vi "PTv3.0.vi"(8 "error in":errorcluster) -> ()   [LabVIEW 2017]
doc: "This VI runs in parallel to other tasks. It can contain as many user-defined periodic loops as you need. These can carry out PID or other sorts of timed response."
uses:
  <vilib>/Analysis/baseanly.llb/Mean (DBL).vi
  <vilib>/Rock Robotics/WPI/Utilities/WPI_GetSetVariantRefNum.vi
  <vilib>/Rock Robotics/Network Tables/NT Read Boolean.vi
  Robot Global Data.vi
  <vilib>/Rock Robotics/Network Tables/NT Write Number.vi
  <vilib>/Rock Robotics/Network Tables/NT Write Numeric Array.vi
  <vilib>/Analysis/NI_AALBase.lvlib
panel:
  out "Arrayval":dbl
  out "Accelerations":T1
  out "Avg Y":dbl
  out "Current Joy Y Value":dbl
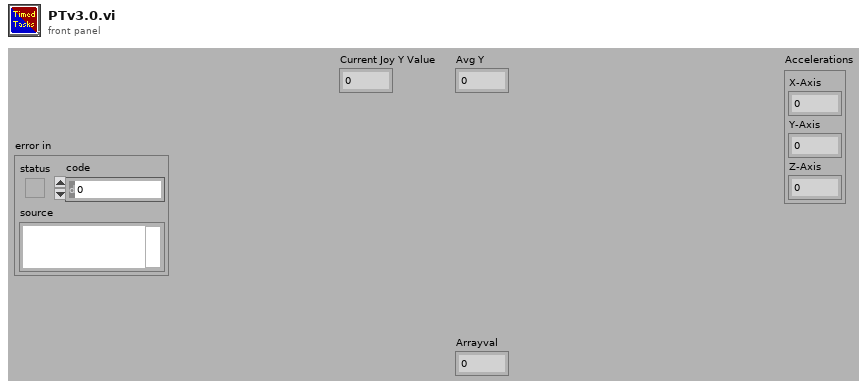
[diagram p1: front panel]
types:
  T1 = cluster{"X-Axis":dbl, "Y-Axis":dbl, "Z-Axis":dbl}
  T2 = typedef "WPI_JoystickDevRef.ctl" = cluster{"Device":T3}
  T3 = typedef "WPI_JoystickDeviceEnum.ctl" = enum16{"USB 0", "USB 1", "USB 2", "USB 3", "USB 4", "USB 5"}
  T4 = typedef "WPI_AccelerometerDevRef.ctl" = cluster{"DevStatus":errorcluster, "Scaling":T5, "Analog Channels":T6, "I2C Bus":T8, "SPI Bus":T9, "Accel Range":T10, "ADXL Axes":T11, "Handle":i32, "Device Address":u8, "Accel Type":enum16{"Analog", "ADXL345 I2C", "ADXL345 SPI", "Internal", "ADXL362 SPI"}}
  T5 = typedef "WPI_AccelerometerScaling.ctl" = cluster{"Gain (VoltsPerG)":dbl, "Center Voltage":dbl}
  T6 = typedef "WPI_AccelerometerAnalogChannels.ctl" = cluster{"X-Axis":T7, "Y-Axis":T7, "Z-Axis":T7}
  T7 = typedef "FPGA_AIChannel.ctl" = enum8{"AI 0", "AI 1", "AI 2", "AI 3", "AI MXP 0", "AI MXP 1", "AI MXP 2", "AI MXP 3", "Invalid"}
  T8 = typedef "i2c_bus.ctl" = enum16{"I2C On-Board", "I2C MXP", "Invalid"}
  T9 = typedef "spi_bus.ctl" = enum16{"SPI On-Board, CS0", "SPI On-Board, CS1", "SPI On-Board, CS2", "SPI On-Board, CS3", "SPI MXP", "Invalid"}
  T10 = typedef "ADXL345 Range.ctl" = u8
  T11 = typedef "WPI_AccelerometerADXL345 Axes.ctl" = cluster{"X-Axis":bool, "Y-Axis":bool, "Z-Axis":bool}
  T12 = typedef "WPI_GyroDevRef.ctl" = cluster{"DevStatus":errorcluster, "Analog Channel":T7, "Gain (VoltsPerDegree/Second)":dbl, "Gyro Type":enum16{"Analog", "XRS450"}, "Handle":i32, "SPI Bus":T9, "Device Found":bool, "Sample Rate":dbl, "Calibrate On Open":bool, "Offset":dbl}
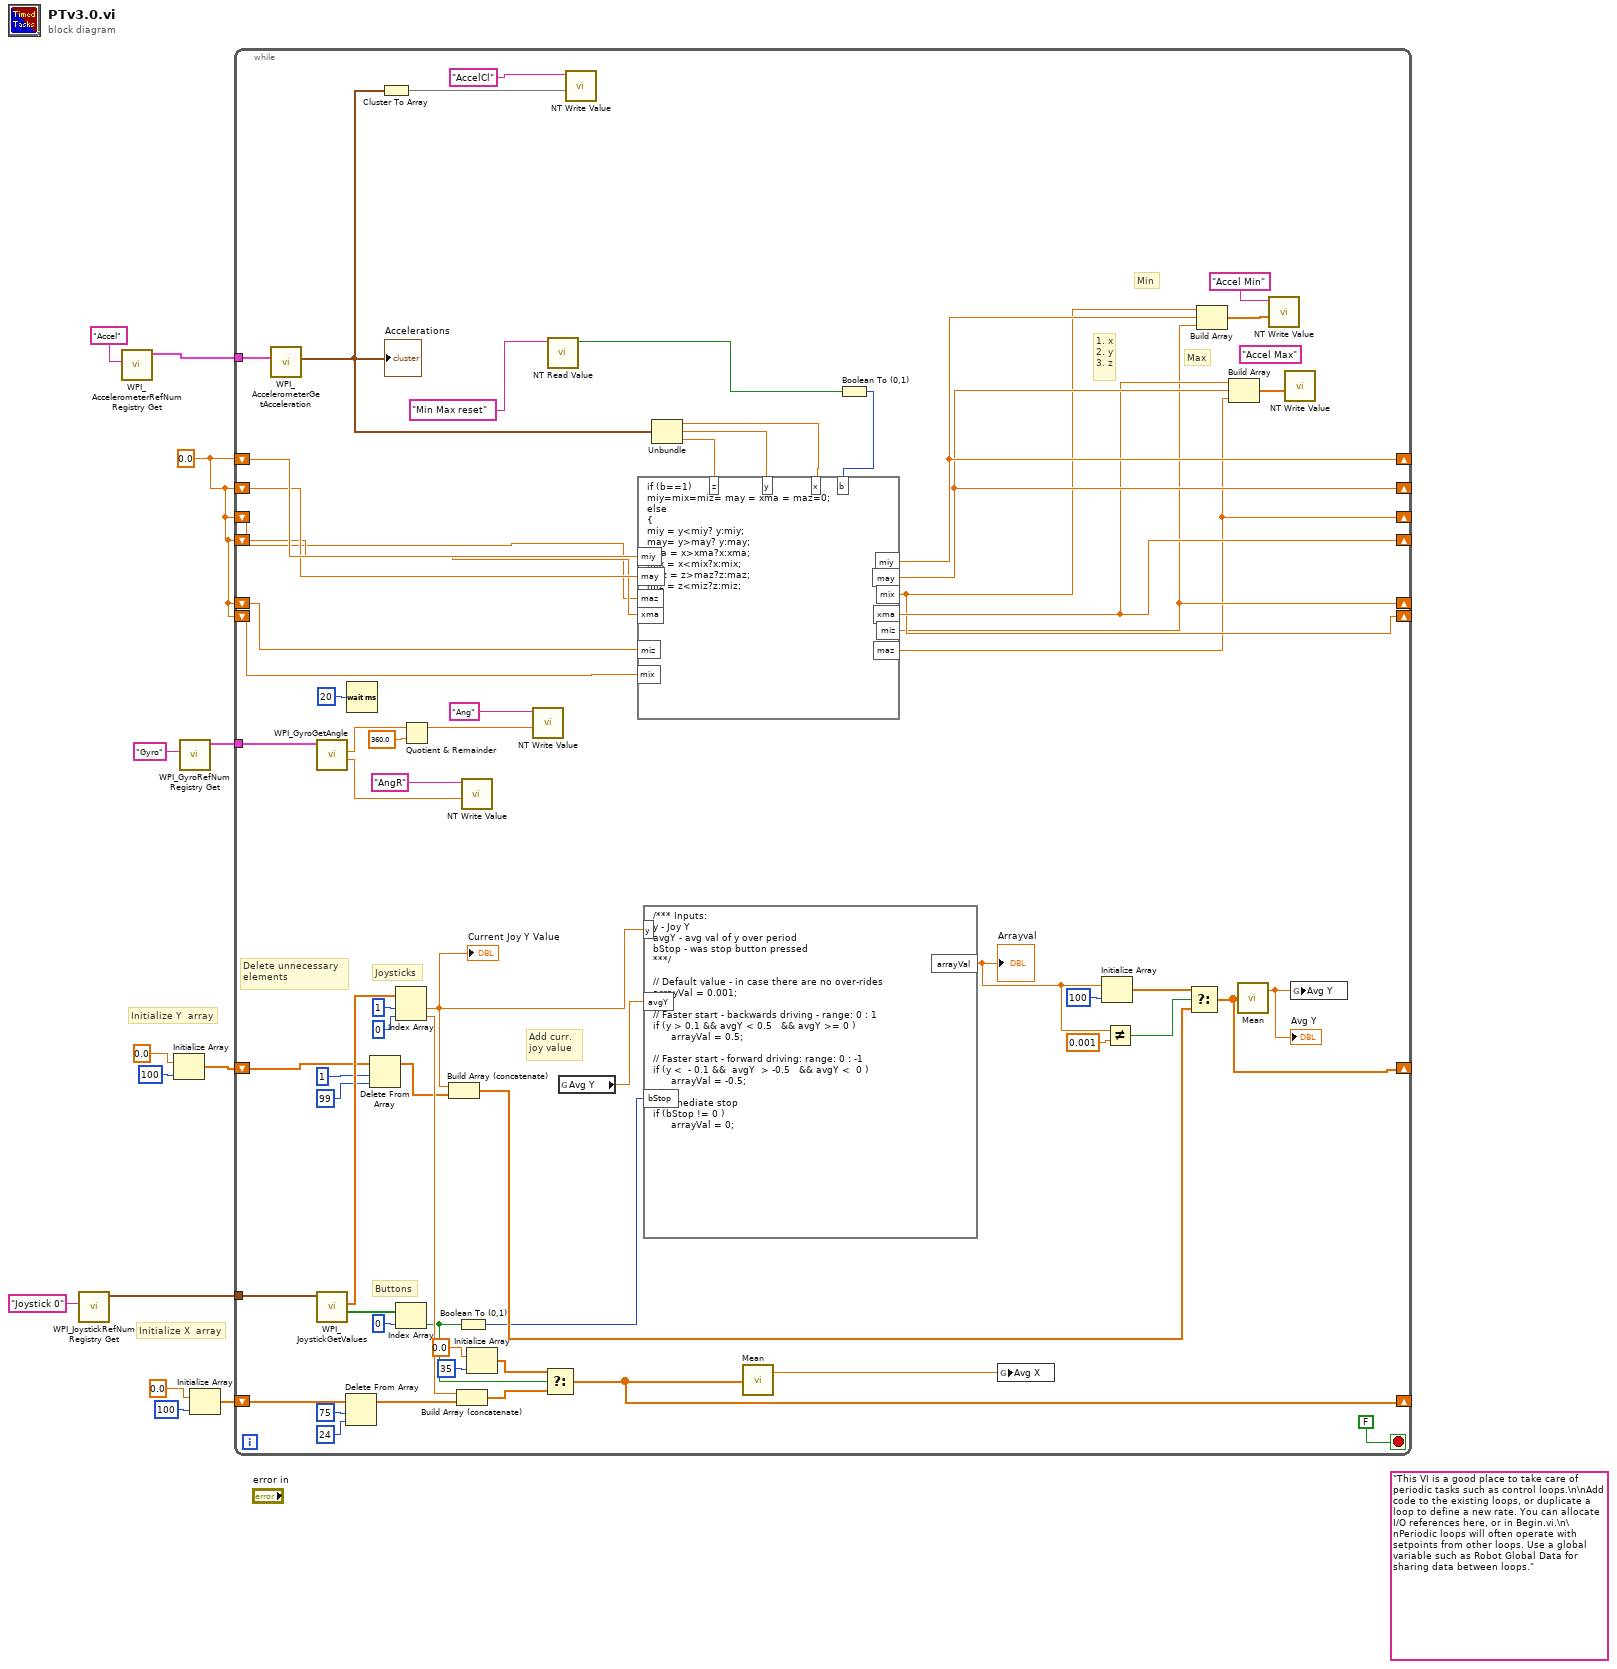
[diagram p0: block diagram]
diagram:
  w1 = 0.0 ("Y-Axis")
  (unwired) "This VI is a good place to take care of periodic tasks such as control loops.\n\nAdd code to the existing loops, or duplicate a loop to define a new rate. You can allocate I/O references here, or in Begin.vi.\n\nPeriodic loops will often operate with setpoints from other loops. Use a global variable such as Robot Global Data for sharing data between loops."
  # "Initialize X  array"
  # "Initialize Y  array"
  n1 = call <vilib>:"WPI_JoystickRefNum Registry Get.vi"("refnum name"="Joystick 0") -> ("JoystickDevRef"=w12:T2)  [unwired: 1 in, 9 out]
  n2 = call <vilib>:"WPI_AccelerometerRefNum Registry Get.vi"("refnum name"="Accel") -> ("AccelerometerDevRef"=w4:T4)  [unwired: 9 in, 1 out]
  n3 = Initialize Array(0.0 ("element"), 100 ("dimension size")) -> (w9:dbl[])
  n4 = call <vilib>:"WPI_GyroRefNum Registry Get.vi"("refnum name"="Gyro") -> ("GyroDevRef"=w2:T12)  [unwired: 9 in, 1 out]
  n5 = Initialize Array(0.0 ("element"), 100 ("dimension size")) -> (w8:dbl[])
  n6 = while {
    tunnel: w12 -> [w78]
    shift-right: [w54] -> _
    shift-left: w9 -> [w75]
    shift-right: [w71] -> _
    shift-left: w8 -> [w66]
    tunnel: w4 -> [w49]
    tunnel: w2 -> [w48]
    shift-right: [w22] -> _
    shift-left: w1 -> [w28]
    shift-right: [w23] -> _
    shift-left: w1 -> [w29]
    shift-right: [w19] -> _
    shift-left: w1 -> [w26]
    shift-right: [w21] -> _
    shift-left: w1 -> [w27]
    shift-right: [w24] -> _
    shift-left: w1 -> [w30]
    shift-right: [w20] -> _
    shift-left: w1 -> [w25]
    stop <- FALSE stop-if-true
    (unwired) "Accel Max" ("Name")
    # "1. x\n2. y\n3. z"
    # "Max"
    # "Min"
    # "Add curr. \njoy value"
    # "Delete unnecessary \nelements"
    # "Joysticks"
    # "Buttons"
    n7 = call <vilib>:"WPI_AccelerometerGetAcceleration.vi"("AccelerometerDevRef"=w49) -> ("Accelerations"=w39:T1)  [unwired: 8 in, 2 out]
    "Accelerations" <- w39
    n8 = call <vilib>:"WPI_GyroGetAngle.vi"("GyroDevRef"=w48) -> ("Angular Rate"=w46:dbl, "Angle"=w41:dbl)  [unwired: 6 in, 3 out]
    n9 = call <vilib>:"WPI_JoystickGetValues.vi"("JoystickDevRef"=w78) -> ("Buttons"=w74:bool[], "Axes"=w77:dbl[])  [unwired: 6 in, 3 out]
    n10 = Delete From Array(array=w66, length=75, index=24) -> (array with subset deleted=w67:dbl[])  [unwired: 1 out]
    n11 = Wait (ms)(milliseconds to wait=u32 20) -> ()  [unwired: 1 out]
    n12 = Delete From Array(array=w75, length=1, index=99) -> (array with subset deleted=w59:dbl[])  [unwired: 1 out]
    n13 = Cluster To Array(cluster=w39) -> (array=w47:dbl[])
    n14 = Index Array(array=w77, index #1=1 ("index"), index #2=0 ("index")) -> (element #1=w50:dbl, element #2=w64:dbl)
    "Current Joy Y Value" <- w50
    n15 = Index Array(array=w74, index=0) -> (element=w55:bool)
    n16 = Quotient & Remainder(x=w41, y=360.0) -> (x-y*floor(x/y)=w40:dbl)  [unwired: 1 out]
    n17 = Build Array (concatenate)(w50, w59) -> (w58:dbl[])
    n18 = Build Array (concatenate)(w64, w67) -> (w65:dbl[])
    n19 = Boolean To (0,1)(Boolean=w55) -> (0, 1=w56:i16)
    n20 = call-poly <vilib>:"NT Write Value.vi"("Numeric"=w46, "Name"="AngR") -> ()  [unwired: 9 in, 1 out]
    n21 = Initialize Array(0.0 ("element"), 35 ("dimension size")) -> (w70:dbl[])
    n22 = call-poly <vilib>:"NT Write Value.vi"("Numeric"=w40, "Name"="Ang") -> ()  [unwired: 9 in, 1 out]
    n23 = Select(t=w70, s=w55, f=w65) -> (s? t:f=w71:dbl[])
    n24 = call-poly <vilib>:"NT Read Value.vi"("Name"="Min Max reset") -> ("Boolean"=w18:bool)  [unwired: 9 in, 1 out]
    n25 = global read "Robot Global Data.vi" "Avg Y"() -> (w57:dbl)
    n26 = call-poly <vilib>:"NT Write Value.vi"("Numeric Array"=w47, "Name"="AccelCl") -> ()  [unwired: 9 in, 1 out]
    n27 = formula code="/*** Inputs:\ny - Joy Y\navgY - avg val of y over period\nbStop - was stop button pressed\n***/\n\n// Default value - in case there are no over-rides\narrayVal = 0.001;\n\n// Faster start - backwards driving - range: 0 : 1\nif (y > 0.1 && avgY < 0.5   && avgY >= 0 )\n      arrayVal = 0.5;\n\n// Faster start - forward driving: range: 0 : -1\nif (y <  - 0.1 &&  avgY  > -0.5   && avgY <  0 )\n      arrayVal = -0.5;\n\n// Immediate stop\nif (bStop != 0 )\n      arrayVal = 0;"("y"=w50, "avgY"=w57, "bStop"=w56) -> ("arrayVal"=w51:dbl)
    "Arrayval" <- w51
    n28 = Unbundle(w39) -> ("X-Axis"=w33:dbl, "Y-Axis"=w32:dbl, "Z-Axis"=w31:dbl)
    n29 = call-poly <vilib>:"Mean.vi"("X"=w71) -> ("mean"=w38:dbl)  [unwired: 1 out]
    n30 = Boolean To (0,1)(Boolean=w18) -> (0, 1=w17:i16)
    n31 = formula code="if (b==1)\nmiy=mix=miz= may = xma = maz=0;\nelse \n{\nmiy = y<miy? y:miy;\nmay= y>may? y:may;\nxma = x>xma?x:xma;\nmix = x<mix?x:mix;\nmaz = z>maz?z:maz;\nmiz = z<miz?z:miz;\n}"("miy"=w30, "may"=w29, "x"=w33, "y"=w32, "z"=w31, "mix"=w27, "xma"=w28, "miz"=w25, "maz"=w26, "b"=w17) -> ("miy"=w24:dbl, "may"=w23:dbl, "mix"=w21:dbl, "xma"=w22:dbl, "miz"=w20:dbl, "maz"=w19:dbl)
    n32 = global write "Robot Global Data.vi" "Avg X"(w38) -> ()
    n33 = Initialize Array(w51, 100 ("dimension size")) -> (w61:dbl[])
    n34 = Not Equal?(x=w51, y=0.001) -> (x != y?=w53:bool)
    n35 = Select(t=w61, s=w53, f=w58) -> (s? t:f=w54:dbl[])
    n36 = Build Array(w21, w24, w20) -> (w15:dbl[])
    n37 = Build Array(w22, w23, w19) -> (w16:dbl[])
    n38 = call-poly <vilib>:"Mean.vi"("X"=w54) -> ("mean"=w37:dbl)  [unwired: 1 out]
    "Avg Y" <- w37
    n39 = call-poly <vilib>:"NT Write Value.vi"("Numeric Array"=w15, "Name"="Accel Min") -> ()  [unwired: 9 in, 1 out]
    n40 = call-poly <vilib>:"NT Write Value.vi"("Numeric Array"=w16) -> ()  [unwired: 10 in, 1 out]
    n41 = global write "Robot Global Data.vi" "Avg Y"(w37) -> ()
  }
